vi "solar Destroy.vi"(8 "error in (no error)":errorcluster, 9 "Shutdown Timeout (60 sec)":u32=60, 11 "solar in":refnum<class "solar.lvclass">) -> (0 "error out":errorcluster)   [LabVIEW 2018, in "solar.lvclass"]
doc: "This destroys and shutdown the target. Use the optional override VI to teardown this target's references before shutting down. If this is the main target, this waits until all child targets shutdown (i.e. release their queues) before closing the SOLAR user interface, destroying the remaining references and exit the application."
uses:
  solar.lvclass
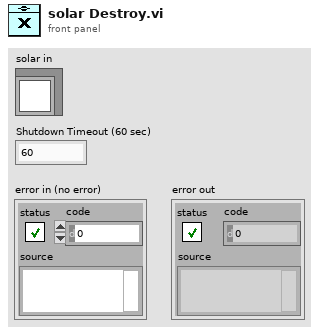
[diagram p1: front panel]
types:
  T1 = typedef "solar_ctl SOLAR Refnum.ctl" = refnum<k1>
  T2 = typedef "solar_ctl SOLAR Global.ctl" = cluster{"Targets":T3[], "AppDir":path, "solar.ini":path, "ConfigsDir":path, "CosmosDir":path, "LogsDir":path, "ExePath":path, "ExeVersion":string, "PartNum":string, "AppSetup":string, "Title":string, "Main.ini":path, "Temp.ini":path, "vSOLAR":string, "Splash.png":string, "SplashWait":i32, "SOLARUE":refnum<user-event>, "VoyagerRefnum":T4, "QTimerRefnum":T5}
  T3 = typedef "solar_ctl Target Global.ctl" = cluster{"Target":string, "Q":refnum<queue>, "UE":refnum<user-event>, "VI":refnum<vi>, "Menu":refnum<k9>, "Data":refnum<data-value>, "Attributes":variant}
  T4 = typedef "solar_voy_ctl Voyager Refnum.ctl" = refnum<k1>
  T5 = typedef "solar_qtimer_ctl Refnum.ctl" = refnum<k1>
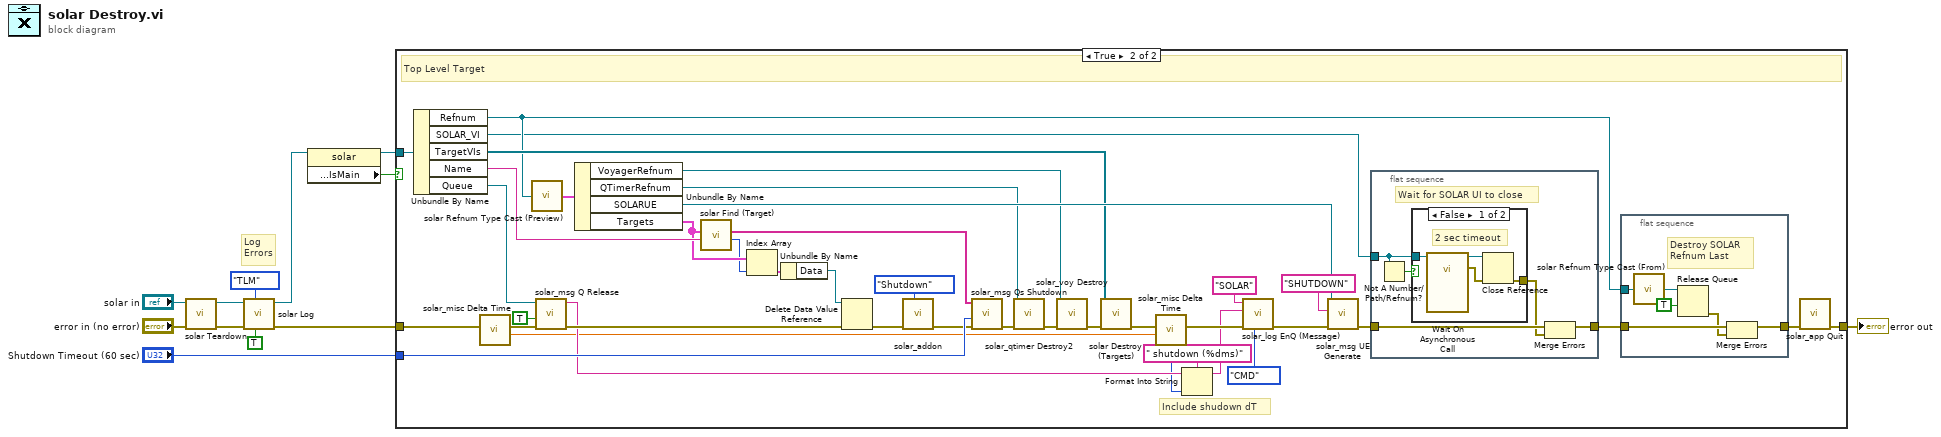
[diagram p0: block diagram]
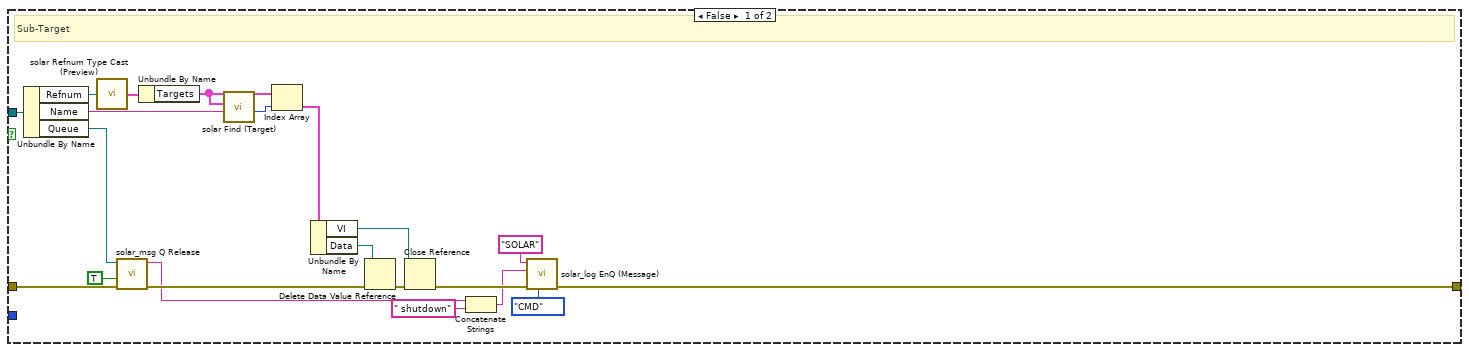
[diagram p2: hidden frame]
diagram:
  # "Log\nErrors"
  n1 = call-dynamic "solar Teardown.vi"("error in (no error)"="error in (no error)", "solar in"="solar in") -> ("error out"=w8:errorcluster, "solar out"=w7:refnum<class "solar.lvclass">)  [unwired: 8 in]
  n2 = call "solar Log.vi"("Clear Error? (T)"=TRUE, "Type (TLM)"=enum8{"CMD", "TLM"}."TLM", "error in (no error)"=w8, "solar in"=w7) -> ("error out"=w4:errorcluster, "solar out"=w6:refnum<class "solar.lvclass">)  [unwired: 6 in]
  n3 = property class="solar"(reference=w6) -> (reference out=w2:refnum<class "solar.lvclass">, "Accessors:Main.IsMain"=w10:bool)  [unwired: 1 in, 1 out]
  n4 = case shown="True" w10 {
    tunnel: w4 -> [w19 w50]
    tunnel: [w18 w34] -> w3
    tunnel: w2 -> [w17 w62]
    tunnel: "Shutdown Timeout (60 sec)" -> [_ w51]
    frame False {
      # "Sub-Target"
      n5 = Unbundle By Name(w17) -> ("Refnum"=w33:T1, "Name"=w31:string, "Queue"=w20:refnum<queue>)
      n6 = call "solar Refnum Type Cast (Preview).vi"("Refnum"=w33) -> ("SOLAR"=w32:T2)  [unwired: 8 in]
      n7 = call "solar_msg Q Release.vi"("error in (no error)"=w19, "Force Destroy? (F)"=TRUE, "Queue"=w20) -> ("error out"=w25:errorcluster, "Queue Name"=w15:string)  [unwired: 6 in, 1 out]
      n8 = Unbundle By Name(w32) -> ("Targets"=w30:T3[])
      n9 = call "solar Find (Target).vi"("Target"=w31, "Targets"=w30) -> ("Target Index"=w29:i32)  [unwired: 8 in, 1 out]
      n10 = Index Array(array=w30, index=w29) -> (element=w28:T3)
      n11 = Unbundle By Name(w28) -> ("VI"=w23:refnum<vi>, "Data"=w26:refnum<data-value>)
      n12 = Delete Data Value Reference(data value reference=w26, error in=w25) -> (error out=w24:errorcluster)  [unwired: 1 out]
      n13 = Close Reference(reference=w23, error in (no error)=w24) -> (error out=w22:errorcluster)
      n14 = Concatenate Strings(w15, " shutdown" ("string")) -> (w13:string)
      n15 = call "solar_log EnQ (Message).vi"("Type (CMD)"=enum8{"CMD", "TLM"}."CMD", "error in (no error)"=w22, "MSG"=w13, "Target"="SOLAR") -> ("error out"=w18:errorcluster)  [unwired: 7 in]
    }
    frame True {
      # "Include shudown dT"
      # "Top Level Target"
      n16 = Unbundle By Name(w62) -> ("Refnum"=w59:T1, "SOLAR_VI"=w58:refnum<vi>, "TargetVIs"=w61:refnum<vi>[], "Name"=w70:string, "Queue"=w64:refnum<queue>)
      n17 = call "solar_misc Delta Time.vi"("error in (no error)"=w50) -> ("error out"=w49:errorcluster, "Current Time (sec)"=w35:dbl)  [unwired: 6 in, 1 out]
      n18 = call "solar Refnum Type Cast (Preview).vi"("Refnum"=w59) -> ("SOLAR"=w71:T2)  [unwired: 8 in]
      n19 = call "solar_msg Q Release.vi"("error in (no error)"=w49, "Force Destroy? (F)"=TRUE, "Queue"=w64) -> ("error out"=w48:errorcluster, "Queue Name"=w39:string)  [unwired: 6 in, 1 out]
      n20 = Unbundle By Name(w71) -> ("VoyagerRefnum"=w65:T4, "QTimerRefnum"=w60:T5, "SOLARUE"=w66:refnum<user-event>, "Targets"=w69:T3[])
      n21 = call "solar Find (Target).vi"("Target"=w70, "Targets"=w69) -> ("Target Index"=w68:i32, "Target Names"=w52:string[])  [unwired: 8 in]
      n22 = Index Array(array=w69, index=w68) -> (element=w67:T3)
      n23 = Unbundle By Name(w67) -> ("Data"=w63:refnum<data-value>)
      n24 = Delete Data Value Reference(data value reference=w63, error in=w48) -> (error out=w47:errorcluster)  [unwired: 1 out]
      n25 = call "solar_addon.vi"("Action (Launch)"=enum8{"Launch", "Initialize", "Shutdown"}."Shutdown", "error in (no error)"=w47) -> ("error out"=w46:errorcluster)  [unwired: 8 in, 1 out]
      n26 = call "solar_msg Qs Shutdown.vi"("error in (no error)"=w46, "sec Timeout (60)"=w51, "Queue Names"=w52) -> ("error out"=w45:errorcluster)  [unwired: 7 in, 1 out]
      n27 = call "solar_qtimer Destroy2.vi"("error in (no error)"=w45, "QTimer Refnum"=w60) -> ("error out"=w44:errorcluster)  [unwired: 9 in]
      n28 = call "solar_voy Destroy.vi"("error in (no error)"=w44, "Voyager Refnum"=w65) -> ("error out"=w43:errorcluster)  [unwired: 9 in]
      n29 = call "solar Destroy (Targets).vi"("error in (no error)"=w43, "TargetVIs"=w61) -> ("error out"=w41:errorcluster)  [unwired: 9 in]
      n30 = call "solar_misc Delta Time.vi"("error in (no error)"=w41, "Previous Time (sec)"=w35) -> ("error out"=w40:errorcluster, "Delta (ms)"=w36:u32)  [unwired: 5 in, 1 out]
      n31 = Format Into String(format string=" shutdown (%dms)", initial string=w39, w36) -> (resulting string=w38:string)  [unwired: 1 in, 1 out]
      n32 = call "solar_log EnQ (Message).vi"("Type (CMD)"=enum8{"CMD", "TLM"}."CMD", "error in (no error)"=w40, "MSG"=w38, "Target"="SOLAR") -> ("error out"=w53:errorcluster)  [unwired: 7 in]
      n33 = call "solar_msg UE Generate.vi"("error in (no error)"=w53, "CMD (Last)"="SHUTDOWN" ("Packet"), "UserEvent in"=w66) -> ("error out"=w56:errorcluster)  [unwired: 7 in, 1 out]
      n34 = flat-sequence {
        tunnel: w58 -> [w76]
        tunnel: [w78] -> w42
        tunnel: w56 -> [w79]
        frame #0 {
          # "Wait for SOLAR UI to close"
          n35 = Not A Number/Path/Refnum?(number/path/refnum=w76) -> (NaN/Path/Refnum?=w75:bool)
          n36 = case shown="False" w75 {
            tunnel: w76 -> [w83 _]
            tunnel: [w80 _] -> w77
            frame False {
              # "2 sec timeout"
              n37 = call-by-ref "Wait On Asynchronous Call"(reference=w83) -> (reference out=w82:refnum<vi>, error out=w81:errorcluster)  [unwired: 13 in]
              n38 = Close Reference(reference=w82, error in (no error)=w81) -> (error out=w80:errorcluster)
            }
            frame True {
            }
          }
          n39 = Merge Errors(w79, w77) -> (w78:errorcluster)
        }
      }
      n40 = flat-sequence {
        tunnel: w42 -> [w89]
        tunnel: [w85] -> w73
        tunnel: w59 -> [w88]
        frame #0 {
          # "Destroy SOLAR \nRefnum Last"
          n41 = call "solar Refnum Type Cast (From).vi"("Refnum"=w88) -> ("SOLAR"=w87:refnum<queue>)
          n42 = Release Queue(queue=w87, force destroy? (F)=TRUE) -> (error out=w84:errorcluster)  [unwired: 1 in, 2 out]
          n43 = Merge Errors(w89, w84) -> (w85:errorcluster)
        }
      }
      n44 = call "solar_app Quit.vi"("error in (no error)"=w73) -> ("error out"=w34:errorcluster)  [unwired: 10 in]
    }
  }
  "error out" <- w3
